vi "transmitRFID cw_query.vi"() -> ()   [LabVIEW 2015]
uses:
  <instrlib>/niUSRP/niUSRP Write Tx Data (CDB).vi
panel:
  in  "query":bool
  out "ACK Entered":bool
  out "RFID Pushed":bool
  out "error out":errorcluster
  in  "Parameters Query":T1 {"Session" items=["S0", "S1", "S2", "S3"]; "Sel" items=["All", "All2", "~SL", "SL"]; "M" items=["M=1", "M=2", "M=4", "M=8"]}
  out "Waveform Magnitude":dbl[](graph)
  out "Loop":i32
  in  "Symbol Rate [Hz]":dbl=500000.0 format="%#_13p"
  in  "Parameters Select":T2={"Target"=7, "Action"=0, "MemBank"=1, "truncate"=FALSE} {"MemBank" items=["00 RFU", "01 EPC", "10 TID", "11 User"]; "Action" items=["000", "001", "010", "011", "100", "101", "110", "111"]; "Target" items=["000 Inventoried (S0)", "001 Inventoried (S1)", "010 Inventoried (S2)", "011 Inventoried (S3)", "100 SL", "101 RFU", "110 RFU", "111 RFU"]}
  in  "Parameters Symbols":T3={"Tari"=8e-06, "PW"=0.5, "factor for \"1\" symbol"=0.5, "RTcal"=2.5, "TRcal"=3.0, "Delimiter"=1.25e-05} {"TRcal" min=1.1 max=3.0 step=0.1; "RTcal" min=2.5 max=3.0 step=0.1; "factor for \"1\" symbol" min=0.5 max=1.0 step=0.1; "PW" min=0.265 max=0.525 step=0.001; "Tari" format="%#_3p"}
  out "coerced IQ rate":dbl=100000.0 format="%#_6p"
  out "carrier frequency":dbl=100000.0 format="%#_6p"
  out "coerced gain":dbl format="%#_6f"
  in  "stop":bool
  in  "IQ rate":dbl=2000000.0 format="%#_6p"
  in  "carrier frequency":dbl=920000000.0 format="%#_6p"
  in  "gain":dbl format="%#_6f"
  in  "tx device names":refnum<k15>="192.168.20.13"
  # "Transmit RFID"
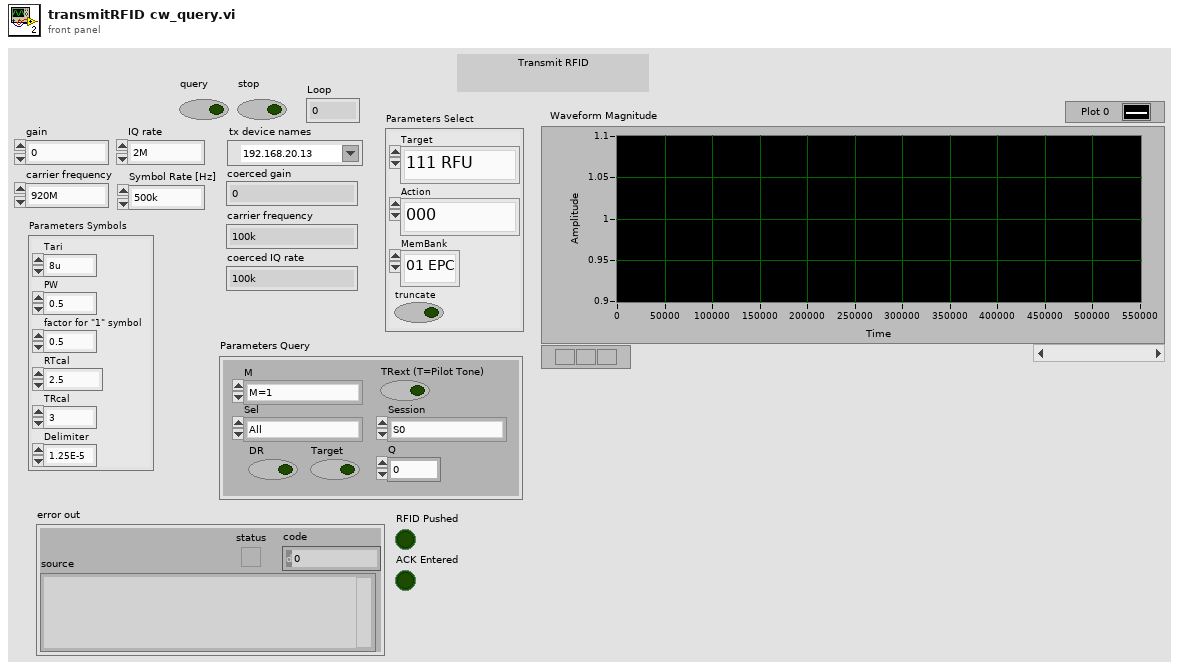
[diagram p1: front panel]
types:
  T1 = cluster{"DR":bool, "M":u16, "TRext (T=Pilot Tone)":bool, "Sel":u16, "Session":u16, "Q":u8, "Target":bool}
  T2 = cluster{"Target":u16, "Action":u16, "MemBank":u16, "truncate":bool}
  T3 = cluster{"Tari":dbl, "PW":dbl, "factor for \"1\" symbol":dbl, "RTcal":dbl, "TRcal":dbl, "Delimiter":dbl}
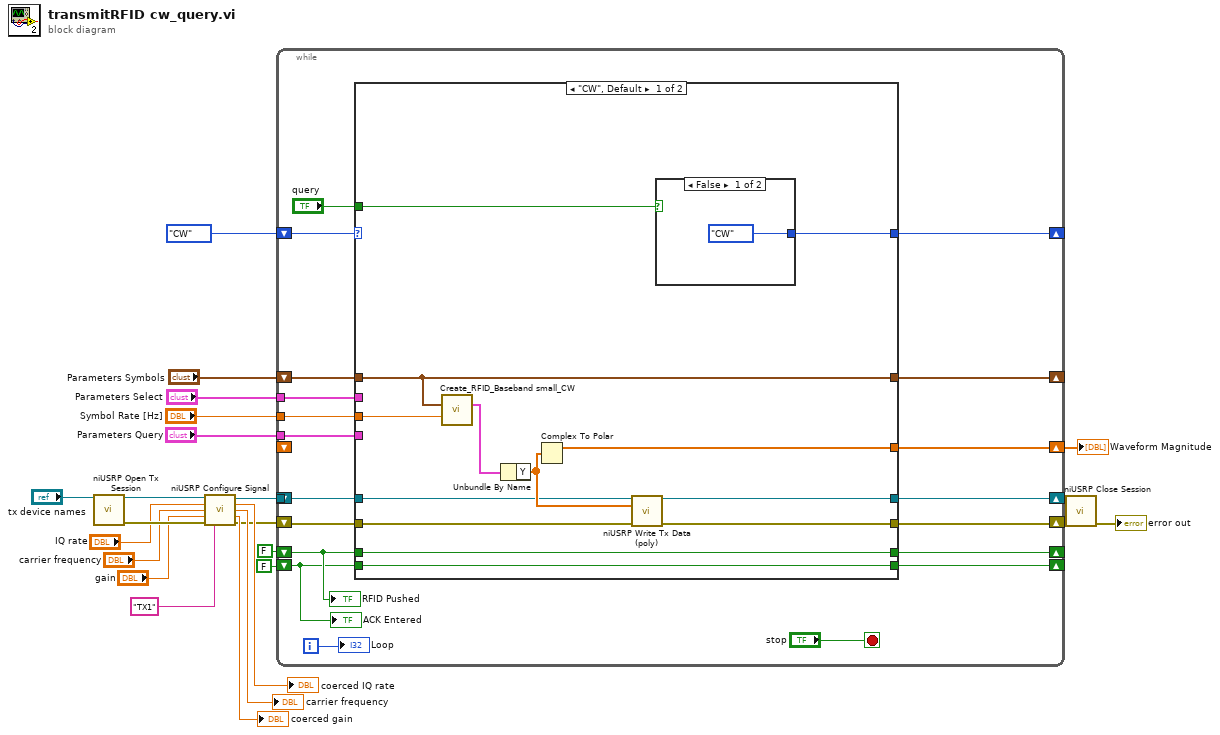
[diagram p0: block diagram]
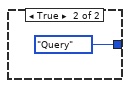
[diagram p2: hidden frame]
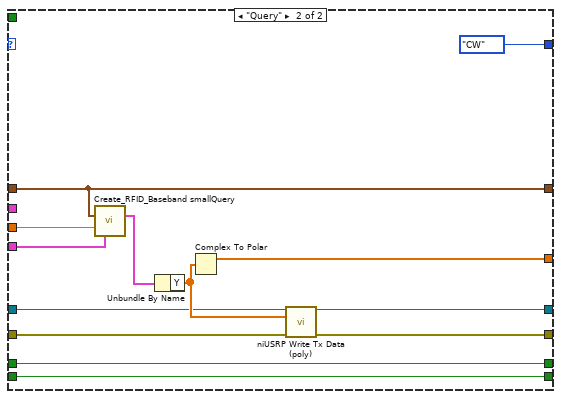
[diagram p3: hidden frame]
diagram:
  n1 = call <instrlib>:"niUSRP Open Tx Session.vi"("device names"="tx device names") -> ("session handle out"=w11:refnum<k15>, "error out"=w23:errorcluster)  [unwired: 13 in]
  n2 = call <instrlib>:"niUSRP Configure Signal.vi"("session handle"=w11, "IQ rate"="IQ rate", "carrier frequency"="carrier frequency", "gain"="gain", "error in (no error)"=w23, "active antenna"="TX1") -> ("session handle out"=w9:refnum<k15>, "coerced IQ rate"=→"coerced IQ rate":dbl, "coerced carrier frequency"=→"carrier frequency":dbl, "coerced gain"=→"coerced gain":dbl, "error out"=w8:errorcluster)  [unwired: 5 in]
  n3 = while {
    tunnel: "Parameters Select" -> [w35]
    tunnel: "Parameters Query" -> [w33]
    tunnel: w9 -> [w40]
    shift-right: [w38] -> w7
    shift-left: w8 -> [w39]
    shift-right: [w37] -> w5
    shift-left: _ -> [_]
    shift-right: [w25] -> _
    shift-left: enum16{"CW", "Query"}."CW" -> [w41]
    shift-right: [w32] -> _
    shift-left: "Parameters Symbols" -> [w36]
    shift-right: [w30] -> _
    shift-left: FALSE -> [w29]
    shift-right: [w28] -> _
    shift-left: FALSE -> [w27]
    shift-right: [w26] -> w1
    shift-left: _ -> [_]
    tunnel: "Symbol Rate [Hz]" -> [w34]
    i -> [w42]
    stop <- "stop" stop-if-true
    n4 = case shown="\"CW\", Default" w41 {
      tunnel: w40 -> [w54 w69]
      tunnel: w39 -> [w53 w68]
      tunnel: [w52 w67] -> w38
      tunnel: [w51 w66] -> w37
      tunnel: w36 -> [w47 w58]
      tunnel: w35 -> [_ _]
      tunnel: w34 -> [w46 w59]
      tunnel: w33 -> [_ w60]
      tunnel: [w47 w58] -> w32
      tunnel: [w50 w65] -> w30
      tunnel: w29 -> [w50 w65]
      tunnel: [w49 w64] -> w28
      tunnel: w27 -> [w49 w64]
      tunnel: [w48 w63] -> w26
      tunnel: [w44 enum16{"CW", "Query"}."CW"] -> w25
      tunnel: "query" -> [w43 _]
      frame "CW", Default {
        n5 = call "Create_RFID_Baseband small_CW.vi"("Parameters Symbols"=w47, "Symbol Rate [Hz]"=w46) -> ("complex waveform"=w45:cluster{"t0":dbl, "dt":dbl, "Y":cdb[]})  [unwired: 12 in, 1 out]
        n6 = Unbundle By Name(w45) -> ("Y"=w55:cdb[])
        n7 = Complex To Polar(r * e^(i*theta)=w55) -> (r=w48:dbl[])  [unwired: 1 out]
        n8 = call-poly <instrlib>:"niUSRP Write Tx Data (poly).vi"("session handle"=w54, "data"=w55, "error in (no error)"=w53) -> ("session handle out"=w51:refnum<k15>, "error out"=w52:errorcluster)  [unwired: 11 in]
        n9 = case shown="False" w43 {
          tunnel: [enum16{"CW", "Query"}."CW" enum16{"CW", "Query"}."Query"] -> w44
          frame False {
          }
          frame True {
          }
        }
      }
      frame "Query" {
        n10 = call "Create_RFID_Baseband smallQuery.vi"("Parameters Symbols"=w58, "Symbol Rate [Hz]"=w59, "Parameters Query"=w60) -> ("complex waveform"=w61:cluster{"t0":dbl, "dt":dbl, "Y":cdb[]})  [unwired: 11 in, 1 out]
        n11 = Unbundle By Name(w61) -> ("Y"=w70:cdb[])
        n12 = Complex To Polar(r * e^(i*theta)=w70) -> (r=w63:dbl[])  [unwired: 1 out]
        n13 = call-poly <instrlib>:"niUSRP Write Tx Data (poly).vi"("session handle"=w69, "data"=w70, "error in (no error)"=w68) -> ("session handle out"=w66:refnum<k15>, "error out"=w67:errorcluster)  [unwired: 11 in]
      }
    }
    "Loop" <- w42
    "RFID Pushed" <- w29
    "ACK Entered" <- w27
  }
  "Waveform Magnitude" <- w1
  n14 = call <instrlib>:"niUSRP Close Session.vi"("session handle"=w5, "error in (no error)"=w7) -> ("error out"=→"error out":errorcluster)  [unwired: 13 in]
